vi "FRCts20_WebMethods_Team_PUT.vi"(7 "LabVIEW Web Service Request":refnum<class "Web Request.lvclass">) -> ()   [LabVIEW 2014, in "FRCts20_WebMethods.lvlib"]
doc: "<B>PUT</B> on the specified <B>team</B> resource\n\n<B>Required XML Data : </B>\n<Team>\n <SWType>[<B>unknown</B>, <B>LabVIEW</B>, <B>Windriver, C++</B>, <B>JavaBeans</B>, <B>Other</B>]</SWType>\n <Division><B>string</B></Division>\n</Team>\n\n<B>Required HTML Post Data : </B>\nSWType: [<B>unknown</B>, <B>LabVIEW</B>, <B>Windriver, C++</B>, <B>JavaBeans</B>, <B>Other</B>]\nDivision: <B>string</B>\n\nhttp://<server address>:<port>/FRCts/team"
uses:
  FRCts20_WebMethods.lvlib
  <vilib>/wsapi/Web Request.lvclass
  Backend/source/VI Source/FRCts20_Backend_API/Team.ctl
  Backend/source/VI Source/FRCts20_Backend_API/ApiReturn.ctl
  Backend/source/VI Source/FRCts20_Backend_API/TeamRoot.ctl
  Backend/source/VI Source/FRCts20_Backend_API/FRCts20_Backend_API_SW.ctl
  Backend/source/VI Source/FRCts20_Backend_API/TeamExtended.ctl
  Backend/source/VI Source/FRCts20_Backend_API/EventRoot.ctl
  Backend/source/VI Source/FRCts20_Backend_API/FRCts20_Backend_API_Command_Team.ctl
  FRCts20_WebMethods_ReadData_Team.vi
  Backend/source/VI Source/FRCts20_Backend_API/FRCts20_Backend_API_Team.vi
  Backend/source/VI Source/FRCts20_Backend_API/FRCts20_Backend_API.lvlib
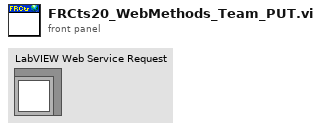
[diagram p1: front panel]
types:
  T1 = typedef "FRCts20_Backend_Engine.lvlib/FRCts20_Backend_API.lvlib/Team.ctl" = cluster{"APIReturn":T2, "TeamRoot":T3, "TeamExtendedData":T5, "Events":T6[]}
  T2 = typedef "FRCts20_Backend_Engine.lvlib/FRCts20_Backend_API.lvlib/ApiReturn.ctl" = string
  T3 = typedef "FRCts20_Backend_Engine.lvlib/FRCts20_Backend_API.lvlib/TeamRoot.ctl" = cluster{"TeamIndex":i32, "TeamNumber":u32, "SoftwareType":T4}
  T4 = typedef "FRCts20_Backend_Engine.lvlib/FRCts20_Backend_API.lvlib/FRCts20_Backend_API_SW.ctl" = string
  T5 = typedef "FRCts20_Backend_Engine.lvlib/FRCts20_Backend_API.lvlib/TeamExtended.ctl" = cluster{"TeamName":string, "ShortTeamName":string, "NickName":string, "RobotName":string, "City":string, "State":string, "Country":string, "RookieYear":u32, "CAN":bool, "Vision":bool, "Kinect":bool, "Avatar":string, "Team ID":u32, "Tags":string}
  T6 = typedef "FRCts20_Backend_Engine.lvlib/FRCts20_Backend_API.lvlib/EventRoot.ctl" = cluster{"EventIndex":i32, "EventName":string, "IsLive":bool, "OpenIssues":i32}
  T7 = typedef "FRCts20_Backend_Engine.lvlib/FRCts20_Backend_API.lvlib/FRCts20_Backend_API_Command_Team.ctl" = string
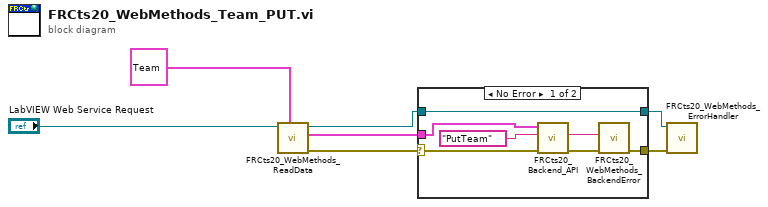
[diagram p0: block diagram]
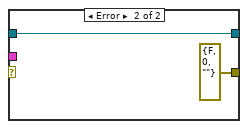
[diagram p2: hidden frame]
diagram:
  n1 = call-poly "FRCts20_WebMethods_ReadData.vi"("TeamRoot"=T1 {"APIReturn"="", "TeamRoot"={"TeamIndex"=0, "TeamNumber"=0, "SoftwareType"=""}, "TeamExtendedData"={"TeamName"="", "ShortTeamName"="", "NickName"="", "RobotName"="", "City"="", "State"="", "Country"="", "RookieYear"=0, "CAN"=FALSE, "Vision"=FALSE, "Kinect"=FALSE, "Avatar"="", "Team ID"=0, "Tags"=""}, "Events"=[]}, "LabVIEW Web Service Request"="LabVIEW Web Service Request") -> ("error out"=w3:errorcluster, "Team Out"=w4:T1, "LabVIEW Web Service Request out"=w2:refnum<class "Web Request.lvclass">)  [unwired: 7 in]
  n2 = case shown="No Error" w3 {
    selector: w3 -> [w8 _]
    tunnel: [w9 errorcluster {"status"=FALSE, "code"=0, "source"=""} ("error out")] -> w6
    tunnel: [w12 w16] -> w5
    tunnel: w2 -> [w12 w16]
    tunnel: w4 -> [w11 _]
    frame No Error {
      n3 = call-poly "FRCts20_Backend_API.vi"("error in (no error)"=w8, "Command"=T7 "PutTeam", "Team In"=w11) -> ("error out"=w14:errorcluster, "Status"=w13:string)  [unwired: 6 in, 1 out]
      n4 = call "FRCts20_WebMethods_BackendError.vi"("error in (no error)"=w14, "Status"=w13) -> ("error out"=w9:errorcluster)  [unwired: 8 in, 1 out]
    }
    frame Error {
    }
  }
  n5 = call "FRCts20_WebMethods_ErrorHandler.vi"("error in"=w6, "LabVIEW Web Service Request"=w5) -> ()  [unwired: 8 in, 2 out]
